vi "Task Loop.vi"(8 "error in (no error)":errorcluster, 11 "SimTask in":refnum<class "SimTask.lvclass">) -> (0 "error out":errorcluster)   [LabVIEW 2020, in "VolatusDemo.lvlib" / "SimTask.lvclass"]
uses:
  SimTask.lvclass
  C:/dev/lv20CE/relink/lv-volatus/Volatus/Task/Task.lvclass
  SimTask.lvclass/SimTask.ctl
  VolatusDataLogger/DataLoggerAPI/DataLoggerAPI.lvclass/DataLoggerAPI.ctl
  VolatusDataLogger/DataLogger Messages/New Data Msg/New Data Msg.lvclass/New Data Msg.ctl
  <vilib>/ActorFramework/Message Enqueuer/Message Enqueuer.lvclass/Message Enqueuer.ctl
  Volatus/Task/Task.lvclass/Task.ctl
  Volatus/TelemetryAPI/TelemetryAPI.lvclass/TelemetryAPI.ctl
  Volatus/Event API/EventAPI.lvclass/EventAPI.ctl
  Volatus/EventHandler Messages/Handle Event Msg/Handle Event Msg.lvclass/Handle Event Msg.ctl
  VolatusDataLogger/DataLogger Messages/New Data Msg/Send New Data.vi
  <vilib>/ActorFramework/Message Enqueuer/Enqueue.vi
  Volatus/Event API/Report Event.vi
  Volatus/EventHandler Messages/Handle Event Msg/Send Handle Event.vi
  lv-vecto/Vecto/Group/Group.lvclass
  C:/dev/lv20CE/relink/lv-vecto/Vecto/GroupAbstract/GroupAbstract.lvclass
  VolatusDataLogger/DataLogger Messages/New Data Msg/New Data Msg.lvclass
  C:/Program Files (x86)/National Instruments/LabVIEW 2020/vi.lib/ActorFramework/Message/Message.lvclass
  Volatus/EventHandler Messages/Handle Event Msg/Handle Event Msg.lvclass
  <vilib>/ActorFramework/Message Priority Queue/Priority Enqueue.vi
  Volatus/Task/Task.lvclass
  VolatusDataLogger/DataLoggerAPI/DataLoggerAPI.lvclass
  C:/Program Files (x86)/National Instruments/LabVIEW 2020/vi.lib/ActorFramework/Actor/Actor.lvclass
  C:/dev/lv20CE/relink/lv-volatus/Volatus/TaskStateHandler/TaskStateHandler.lvclass
  C:/dev/lv20CE/relink/lv-volatus/Volatus/VectoMessageHandler/VectoMessageHandler.lvclass
  C:/dev/lv20CE/relink/lv-volatus/VolatusDemo/SimTask/SimTask.lvclass
  C:/dev/lv20CE/relink/lv-vecto/Vecto/Group/Group.lvclass
panel:
  in  "E":dbl(slide) scale=0.0..100.0
  in  "D":dbl(slide) scale=0.0..100.0
  in  "C":dbl(slide) scale=0.0..100.0
  in  "B":dbl(slide) scale=0.0..100.0
  in  "A":dbl(slide) scale=0.0..100.0
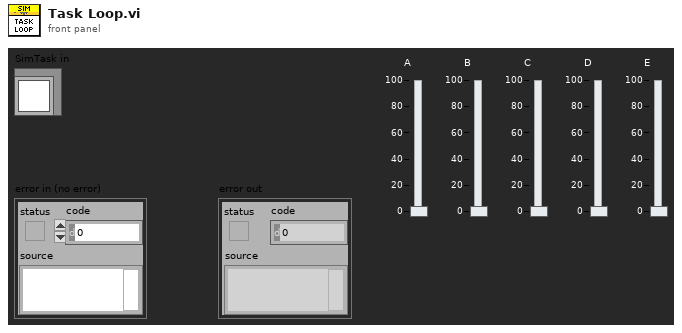
[diagram p1: front panel]
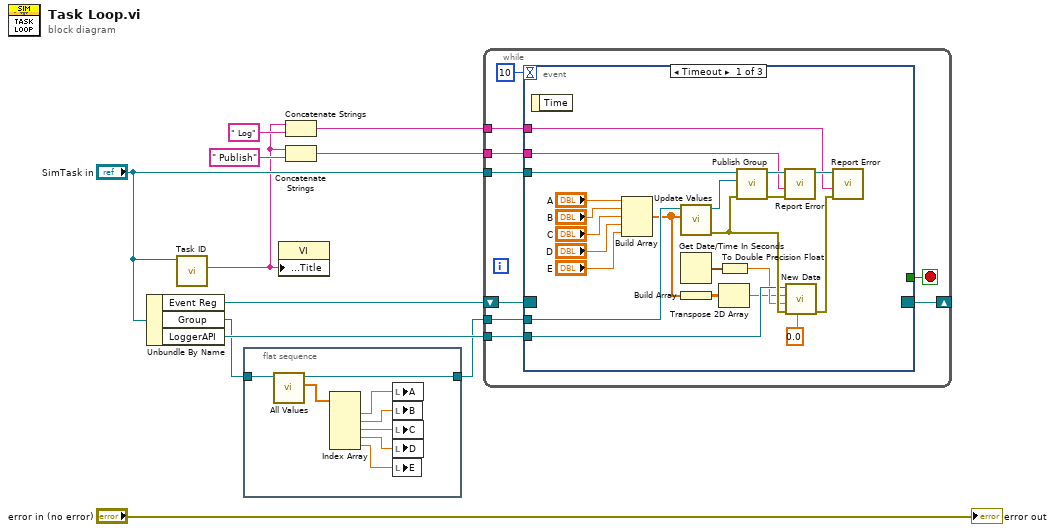
[diagram p0: block diagram]
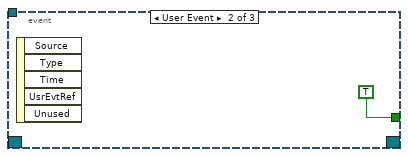
[diagram p2: hidden frame]
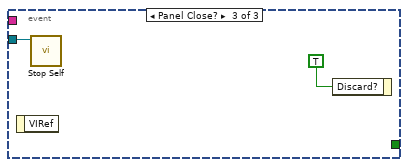
[diagram p3: hidden frame]
diagram:
  n1 = Unbundle By Name("SimTask in") -> ("Event Reg"=w10:refnum<event-registration>, "Group"=w1:refnum<class "Group.lvclass">, "LoggerAPI"=w7:refnum<class "DataLoggerAPI.lvclass">)
  n2 = call-dynamic "Task ID.vi"("Task in"="SimTask in") -> ("Task ID"=w3:string)  [unwired: 8 in, 2 out]
  n3 = flat-sequence {
    tunnel: [w18] -> w2
    tunnel: w1 -> [w19]
    frame #0 {
      n4 = call "All Values.vi"("Group in"=w19) -> ("Scaled"=w17:dbl[], "Group out"=w18:refnum<class "Group.lvclass">)  [unwired: 6 in, 3 out]
      n5 = Index Array(array=w17) -> (element #1=w14:dbl, element #2=w15:dbl, element #3=w16:dbl, element #4=w13:dbl, element #5=w12:dbl)  [unwired: 5 in]
      n6 = local write "A"(w14) -> ()
      n7 = local write "B"(w15) -> ()
      n8 = local write "C"(w16) -> ()
      n9 = local write "D"(w13) -> ()
      n10 = local write "E"(w12) -> ()
    }
  }
  n11 = property class="VI"("Front Panel.Title"=w3) -> ()  [unwired: 2 in, 2 out]
  n12 = Concatenate Strings(w3, " Log" ("string")) -> (w5:string)
  n13 = Concatenate Strings(w3, " Publish" ("string")) -> (w8:string)
  n14 = while {
    shift-right: [w27] -> _
    shift-left: w10 -> [w28]
    tunnel: "SimTask in" -> [w24]
    tunnel: w2 -> [w23]
    tunnel: w8 -> [w22]
    tunnel: w7 -> [w21]
    tunnel: w5 -> [w20]
    stop <- w26 stop-if-true
    n15 = event shown="[0] Timeout" {
      selector: w28 -> [_ _ _]
      dyn-events: [_ _ _] -> w27
      timeout: 10 -> [_ _ _]
      tunnel: [_ TRUE _] -> w26
      tunnel: w24 -> [w43 _ w52]
      tunnel: w23 -> [w44 _ _]
      tunnel: w22 -> [w30 _ _]
      tunnel: w21 -> [w39 _ _]
      tunnel: w20 -> [w29 _ _]
      event Timeout {
        n16 = event-data() -> ()  [unwired: 1 in, 1 out]
        n17 = Build Array("A", "B", "C", "D", "E") -> (w38:dbl[])
        n18 = call "Update Values.vi"("Values"=w38, "Group in"=w44) -> ("error out"=w50:errorcluster, "Group out"=w42:refnum<class "Group.lvclass">)  [unwired: 8 in]
        n19 = Get Date/Time In Seconds() -> (seconds since 1Jan1904=w36:timestamp)
        n20 = Build Array(w38) -> (w37:dbl[][])
        n21 = Transpose 2D Array(2D array=w37) -> (transposed array=w31:dbl[][])
        n22 = To Double Precision Float(number=w36) -> (double precision float=w35:dbl)
        n23 = call "Publish Group.vi"("error in (no error)"=w50, "Group"=w42, "Task in"=w43) -> ("error out"=w40:errorcluster, "Task out"=w41:refnum<class "SimTask.lvclass">)  [unwired: 7 in]
        n24 = call "Report Error.vi"("error in (no error)"=w40, "Message"=w30, "Task in"=w41) -> ("Task out"=w33:refnum<class "SimTask.lvclass">)  [unwired: 7 in, 1 out]
        n25 = call "New Data.vi"("dt"=0.0, "error in (no error)"=w50, "t0"=w35, "Data"=w31, "DataLoggerAPI in"=w39) -> ("error out"=w32:errorcluster)  [unwired: 5 in, 1 out]
        n26 = call "Report Error.vi"("error in (no error)"=w32, "Message"=w29, "Task in"=w33) -> ()  [unwired: 7 in, 2 out]
      }
      event User Event {
        n27 = event-data() -> ()  [unwired: 1 in, 5 out]
      }
      event Panel Close? {
        n28 = event-data() -> ()  [unwired: 1 in, 1 out]
        n29 = call "Stop Self.vi"("Task in"=w52) -> ()  [unwired: 9 in, 2 out]
        n30 = event-data("Discard?"=TRUE) -> ()  [unwired: 1 in, 1 out]
      }
    }
  }
  "error out" <- "error in (no error)"
